vi "Control Loop (Read).vi"(6 "ISOBUS address":T3=-1 caption="ISOBUS address (-1)", 8 "error in":errorcluster, 11 "Mercury Reference In":T4) -> (0 "error out":errorcluster, 2 "Loop Details":T2, 3 "Mercury Reference Out":T4, 4 "Valid?":T1)   [LabVIEW 2018, in "Mercury iXX.lvlib" / "Control Loop.lvlib"]
doc: "Read the current loop configuration for the selected temperature device."
uses:
  Control Loop.lvlib
  Mercury Reference.ctl
  Comms Transport Layer.ctl
  Query Dynamic Reference.ctl
  ISOBus Address.ctl
  Mercury iXX.lvlib_Temperature/Loop Cluster.ctl
  Is Valid LED.ctl
  Command Verbs.ctl
  Mercury iXX.lvlib
  Temperature.lvlib
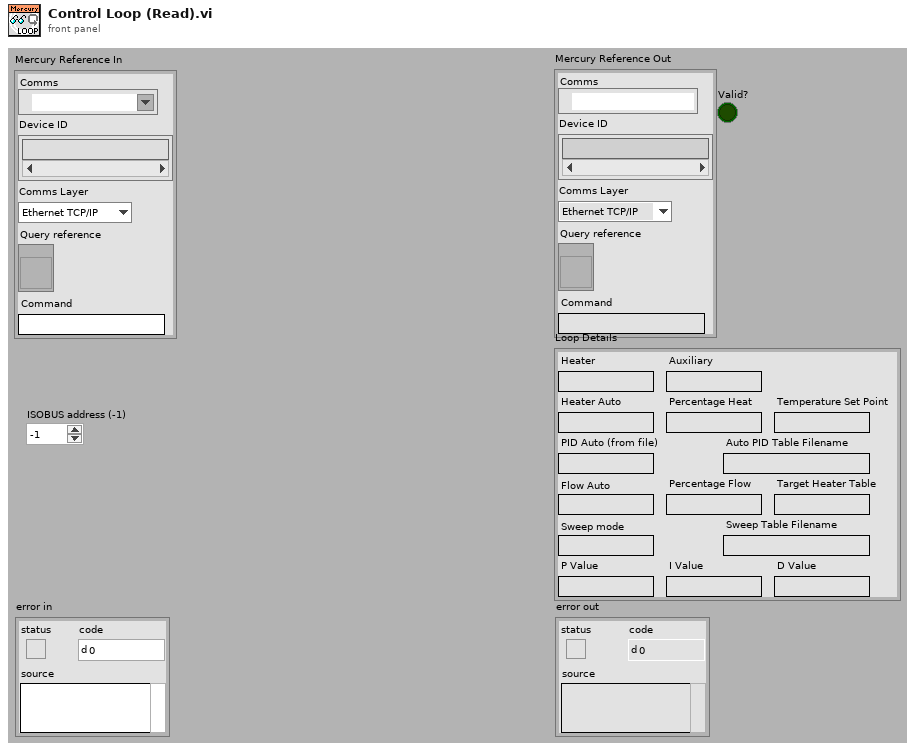
[diagram p1: front panel]
types:
  T1 = typedef "Mercury iXX.lvlib/Is Valid LED.ctl" = bool
  T2 = typedef "Mercury iXX.lvlib/Temperature.lvlib/Loop Cluster.ctl" = cluster{"Heater":string, "Auxiliary":string, "Heater Auto":string, "Percentage Heat":string, "Temperature Set Point":string, "PID Auto (from file)":string, "P Value":string, "I Value":string, "D Value":string, "Auto PID Table Filename":string, "Flow Auto":string, "Target Heater Table":string, "Sweep mode":string, "Sweep Table Filename":string, "Percentage Flow":string}
  T3 = typedef "Mercury iXX.lvlib/ISOBus Address.ctl" = i32
  T4 = typedef "Mercury iXX.lvlib/Mercury Reference.ctl" = cluster{"Comms":refnum<visa-resource-name>, "Device ID":string[], "Comms Layer":T5, "Command":string, "Query reference":T6}
  T5 = typedef "Mercury iXX.lvlib/Comms Transport Layer.ctl" = enum16{"Ethernet TCP/IP", "USB", "ISOBus - RS-232", "GPIB"}
  T6 = typedef "Mercury iXX.lvlib/Query Dynamic Reference.ctl" = refnum<vi>
  T7 = typedef "Mercury iXX.lvlib/Command Verbs.ctl" = string
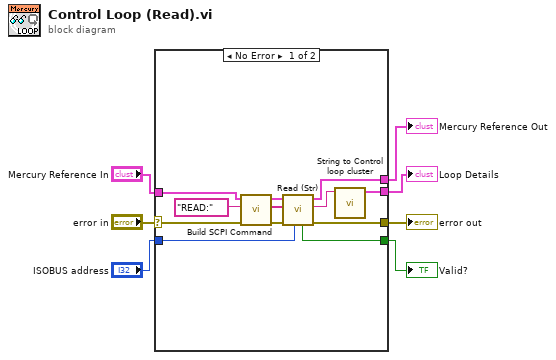
[diagram p0: block diagram]
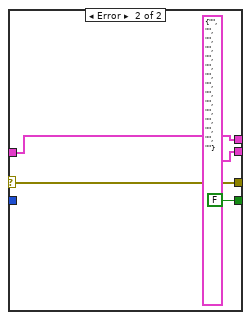
[diagram p2: hidden frame]
diagram:
  n1 = case shown="No Error" "error in" {
    selector: "error in" -> [w14 w22]
    tunnel: "Mercury Reference In" -> [w15 w23]
    tunnel: [w10 w23] -> w5
    tunnel: [w11 w22] -> w7
    tunnel: "ISOBUS address" -> [w13 _]
    tunnel: [w12 FALSE ("Valid?")] -> w6
    tunnel: [w8 T2 {"Heater"="", "Auxiliary"="", "Heater Auto"="", "Percentage Heat"="", "Temperature Set Point"="", "PID Auto (from file)"="", "P Value"="", "I Value"="", "D Value"="", "Auto PID Table Filename"="", "Flow Auto"="", "Target Heater Table"="", "Sweep mode"="", "Sweep Table Filename"="", "Percentage Flow"=""} ("Control Loop")] -> w1
    frame No Error {
      n2 = call "Build SCPI Command.vi"("error in"=w14, "Verb"=T7 "READ:", "Mercury Reference In"=w15) -> ("error out"=w16:errorcluster, "SCPI Message(s)"=w19:string[], "Mercury Reference Out"=w18:T4)  [unwired: 1 in, 5 out]
      n3 = call "Read (Str).vi"("ISOBUS address"=w13, "error in"=w16, "SCPI Message(s)"=w19, "Mercury Reference In"=w18) -> ("error out"=w11:errorcluster, "Response"=w9:string, "Mercury Reference Out"=w10:T4, "Valid?"=w12:T1)  [unwired: 4 out]
      n4 = call "String to Control loop cluster.vi"("Control Loop Details"=w9) -> ("Control Loop"=w8:T2)  [unwired: 10 out]
    }
    frame Error {
    }
  }
  "Mercury Reference Out" <- w5
  "error out" <- w7
  "Loop Details" <- w1
  "Valid?" <- w6
